vi "K_VtodegC.vi"(2 "Voltage (mV)":dbl) -> (0 "Temperature (degC)":sgl)   [LabVIEW 2023]
uses:
  <vilib>/Analysis/NI_AALPro.lvlib
  <vilib>/Analysis/polynomials.llb/Scalar Polynomial Evaluation (DBL).vi
panel:
  out "error":i32
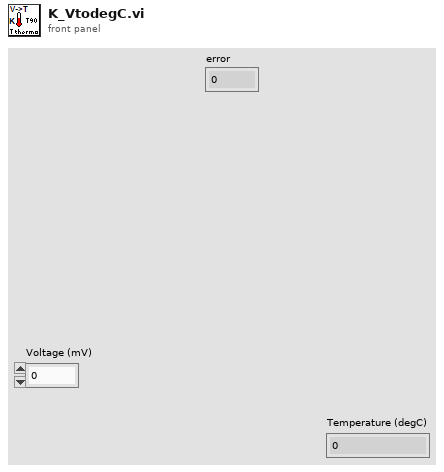
[diagram p1: front panel]
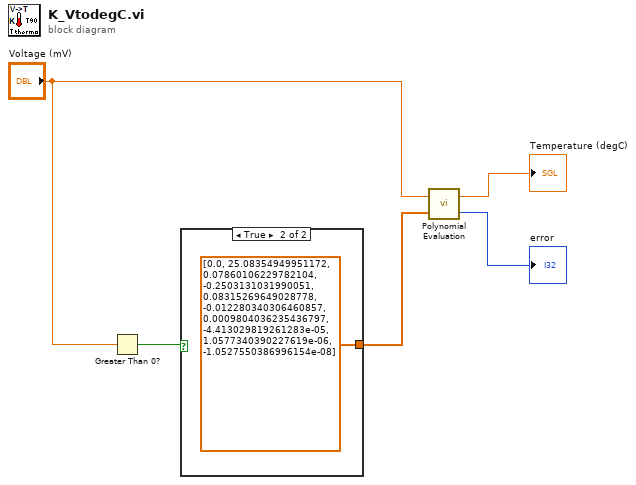
[diagram p0: block diagram]
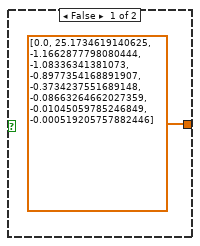
[diagram p2: hidden frame]
diagram:
  n1 = Greater Than 0?(x="Voltage (mV)") -> (x > 0?=w1:bool)
  n2 = case shown="True" w1 {
    tunnel: [sgl[] [0.0, 25.173462, -1.1662878, -1.0833634, -0.8977354, -0.37342376, -0.08663265, -0.010450598, -0.00051920576] ("Coefficinets") sgl[] [0.0, 25.08355, 0.07860106, -0.2503131, 0.0831527, -0.01228034, 0.0009804036, -4.41303e-05, 1.057734e-06, -1.052755e-08] ("Coefficinets")] -> w5
    frame False {
    }
    frame True {
    }
  }
  n3 = call-poly <vilib>:"Polynomial Evaluation.vi"("P(x)"=w5, "a"="Voltage (mV)") -> ("error"=→"error":i32, "P(a)"=→"Temperature (degC)":dbl)
